vi "CLSUIP_IsValidTreeItem.vi"(8 "error in (no error)":errorcluster, 10 "Coords":T1, 11 "TreeRef":refnum<vi>) -> (0 "error out":errorcluster, 1 "Tag":string, 2 "Valid Item Selected?":bool, 3 "TreeRef out":refnum<vi>)   [LabVIEW 2021, in "ChooseImplementation.lvlib"]
uses:
  <resource>/Framework/Providers/LVClassLibrary/ChooseImplementation/ChooseImplementation.lvlib
  <vilib>/Utility/miscctls.llb/LVPoint32TypeDef.ctl
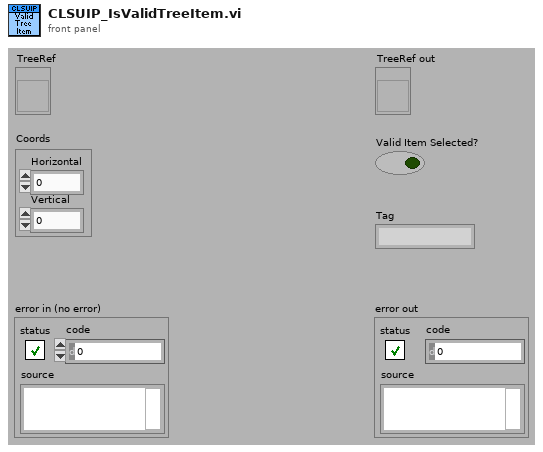
[diagram p1: front panel]
types:
  T1 = typedef "LVPoint32TypeDef.ctl" = cluster{"Horizontal":i32, "Vertical":i32}
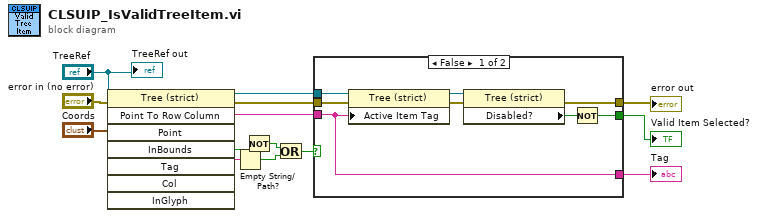
[diagram p0: block diagram]
diagram:
  n1 = invoke class="Tree (strict)" method="Point To Row Column"(reference="TreeRef", error in="error in (no error)", "Point"="Coords") -> (reference out=w7:refnum<vi>, error out=w6:errorcluster, "InBounds"=w11:bool, "Tag"=w5:string)  [unwired: 5 in, 4 out]
  n2 = Empty String/Path?(string/path=w5) -> (empty?=w13:bool)
  n3 = Not(x=w11) -> (.not. x?=w12:bool)
  n4 = Or(x=w12, y=w13) -> (x .or. y?=w8:bool)
  n5 = case shown="False" w8 {
    tunnel: w7 -> [w21 _]
    tunnel: w6 -> [w20 _]
    tunnel: w5 -> [w15 _]
    tunnel: [w16 _] -> w4
    tunnel: [w15 _] -> w3
    tunnel: [w14 _] -> w2
    frame False {
      n6 = property class="Tree (strict)"(reference=w21, error in=w20, "Active Item Tag"=w15) -> (reference out=w19:refnum<vi>, error out=w18:errorcluster)
      n7 = property class="Tree (strict)"(reference=w19, error in=w18) -> (error out=w14:errorcluster, "Disabled?"=w17:bool)  [unwired: 1 out]
      n8 = Not(x=w17) -> (.not. x?=w16:bool)
    }
    frame True {
    }
  }
  "Tag" <- w3
  "Valid Item Selected?" <- w4
  "error out" <- w2
  "TreeRef out" <- "TreeRef"
